vi "Measure number of suns.vi"(8 "error in (no error)":errorcluster) -> (0 "error out":errorcluster, 3 "Number of suns":dbl)   [LabVIEW 2016]
uses:
  <instrlib>/keithley_24xx/Keithley 24XX/Public/Data/Read (Single Point).vi
  <vilib>/Utility/file.llb/Read From Spreadsheet File (string).vi
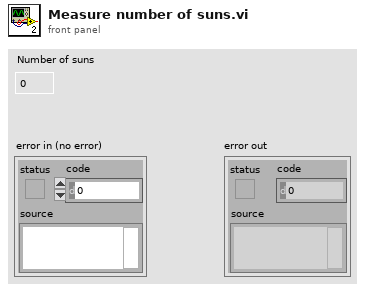
[diagram p1: front panel]
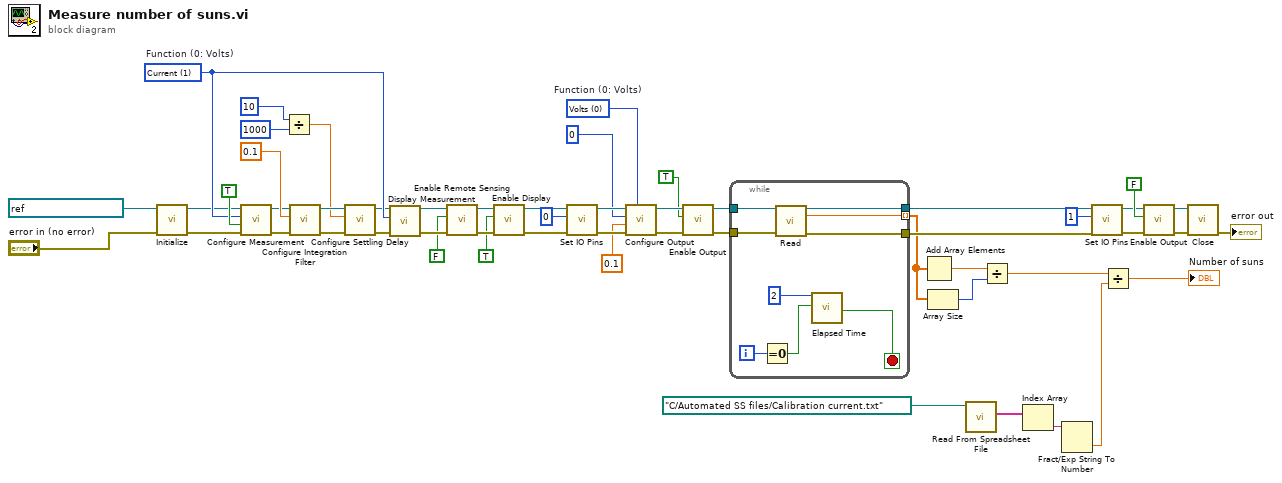
[diagram p0: block diagram]
diagram:
  w15 = u16 0 items=["Volts", "Current", "Resistance"]  # Function (0: Volts)
  w46 = u16 1 items=["Volts", "Current", "Resistance"]  # Function (0: Volts)
  n1 = call <instrlib>:"Initialize.vi"("error in (no error)"="error in (no error)", "VISA resource name"=refnum<visa-resource-name> "GPIB0::24::INSTR") -> ("error out"=w36:errorcluster, "VISA resource name out"=w37:refnum<visa-resource-name>)  [unwired: 3 in, 5 out]
  n2 = call <instrlib>:"Configure Measurement.vi"("error in (no error)"=w36, "Enable Auto Range (T:Enable)"=TRUE, "Function (0: Volts)"=w46, "VISA resource name"=w37) -> ("error out"=w39:errorcluster, "VISA resource name out"=w38:refnum<visa-resource-name>)  [unwired: 6 in]
  n3 = Divide(x=10, y=1000) -> (x/y=w45:dbl)
  n4 = call <instrlib>:"Configure Integration Filter.vi"("error in (no error)"=w39, "Measurement Speed (1 PLC)"=0.1, "VISA resource name"=w38) -> ("error out"=w48:errorcluster, "VISA resource name out"=w47:refnum<visa-resource-name>)  [unwired: 7 in]
  n5 = call <instrlib>:"Configure Settling Delay.vi"("error in (no error)"=w48, "Manual Settling Delay (0 sec)"=w45, "VISA resource name"=w47) -> ("error out"=w43:errorcluster, "VISA resource name out"=w42:refnum<visa-resource-name>)  [unwired: 7 in]
  n6 = call <instrlib>:"Display Measurement.vi"("error in (no error)"=w43, "Displayed Measurement (0: Voltage)"=w46, "VISA resource name"=w42) -> ("error out"=w41:errorcluster, "VISA resource name out"=w40:refnum<visa-resource-name>)  [unwired: 7 in]
  n7 = call <instrlib>:"Enable Remote Sensing.vi"("error in (no error)"=w41, "Enable Remote Sensing (T: Enable)"=FALSE, "VISA resource name"=w40) -> ("error out"=w34:errorcluster, "VISA resource name out"=w35:refnum<visa-resource-name>)  [unwired: 7 in]
  n8 = call <instrlib>:"Enable Display.vi"("error in (no error)"=w34, "Enable Display (T: Enable)"=TRUE ("Enable Output (T: Enable)"), "VISA resource name"=w35) -> ("error out"=w31:errorcluster, "VISA resource name out"=w32:refnum<visa-resource-name>)  [unwired: 7 in]
  n9 = call <instrlib>:"Set IO Pins.vi"("error in (no error)"=w31, "Output Pattern (0)"=0, "VISA resource name"=w32) -> ("error out"=w53:errorcluster, "VISA resource name out"=w52:refnum<visa-resource-name>)  [unwired: 7 in]
  n10 = call <instrlib>:"Configure Output.vi"("Source Mode  (0: Voltage)"=w15, "error in (no error)"=w53, "Compliance  Level (0.1)"=0.1 ("Compliance  Level"), "Output Level (0)"=0, "VISA resource name"=w52) -> ("error out"=w30:errorcluster, "VISA resource name out"=w29:refnum<visa-resource-name>)  [unwired: 5 in]
  n11 = call <instrlib>:"Enable Output.vi"("error in (no error)"=w30, "Enable Output (T: Enable)"=TRUE ("Output (Off)"), "VISA resource name"=w29) -> ("error out"=w25:errorcluster, "VISA resource name out"=w26:refnum<visa-resource-name>)  [unwired: 7 in]
  n12 = while {
    tunnel: w26 -> [w62]
    tunnel: w25 -> [w61]
    tunnel: [w60] -> w20
    tunnel: [w58] -> w10 mode=indexing
    tunnel: [w54] -> w17
    i -> [w57]
    stop <- w59 stop-if-true
    n13 = Equal To 0?(x=w57) -> (x = 0?=w56:bool)
    n14 = call-poly <instrlib>:"Read.vi"("VISA resource name"=w62, "error in (no error)"=w61) -> ("VISA resource name out"=w60:refnum<visa-resource-name>, "Current"=w58:sgl, "error out"=w54:errorcluster)  [unwired: 7 in, 4 out]
    n15 = call "Elapsed Time"("Time Target (s)"=2, "Reset"=w56) -> ("Time has Elapsed"=w59:bool)  [unwired: 10 in, 7 out]
  }
  n16 = Add Array Elements(numeric array=w10) -> (sum=w12:sgl)
  n17 = Array Size(array=w10) -> (size(s)=w9:i32)
  n18 = call-poly <vilib>:"Read From Spreadsheet File.vi"("file path (dialog if empty)"=path "C:/Automated SS files/Calibration current.txt") -> ("first row"=w8:string[])  [unwired: 6 in, 4 out]
  n19 = Divide(x=w12, y=w9) -> (x/y=w11:sgl)
  n20 = Index Array(array=w8) -> (element=w7:string)  [unwired: 1 in]
  n21 = Fract/Exp String To Number(string=w7) -> (number=w6:dbl)  [unwired: 3 in, 1 out]
  n22 = call <instrlib>:"Set IO Pins.vi"("error in (no error)"=w17, "Output Pattern (0)"=1, "VISA resource name"=w20) -> ("error out"=w16:errorcluster, "VISA resource name out"=w21:refnum<visa-resource-name>)  [unwired: 7 in]
  n23 = Divide(x=w11, y=w6) -> (x/y=→"Number of suns":dbl)
  n24 = call <instrlib>:"Enable Output.vi"("error in (no error)"=w16, "Enable Output (T: Enable)"=FALSE ("Output (Off)"), "VISA resource name"=w21) -> ("error out"=w23:errorcluster, "VISA resource name out"=w24:refnum<visa-resource-name>)  [unwired: 7 in]
  n25 = call <instrlib>:"Close.vi"("error in (no error)"=w23, "VISA resource name"=w24) -> ("error out"=→"error out":errorcluster)  [unwired: 9 in]
